vi "PROBE INV SETTING.vi"(8 "INV / NON INV":enum16{"NON INV", "INV"}(ring), 10 "CH":enum16{"CH 1", "CH 2", "CH 3", "CH 4"}(ring), 11 "VISA TSD2014B":refnum<visa-resource-name>="USB0::0x0699::0x0368::C020278::INSTR") -> ()   [LabVIEW 2011]
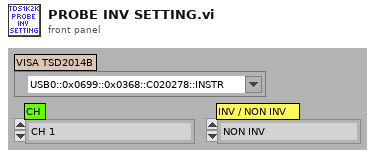
[diagram p1: front panel]
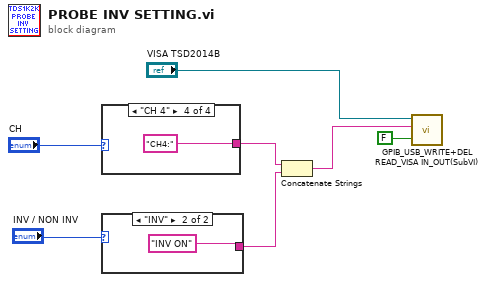
[diagram p0: block diagram]
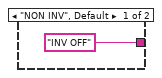
[diagram p2: hidden frame]
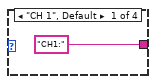
[diagram p3: hidden frame]
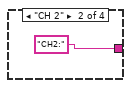
[diagram p4: hidden frame]
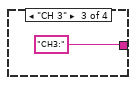
[diagram p5: hidden frame]
diagram:
  n1 = case shown="\"CH 4\"" "CH" {
    tunnel: ["CH1:" "CH2:" "CH3:" "CH4:"] -> w3
    frame "CH 1", Default {
    }
    frame "CH 2" {
    }
    frame "CH 3" {
    }
    frame "CH 4" {
    }
  }
  n2 = case shown="\"INV\"" "INV / NON INV" {
    tunnel: ["INV OFF" "INV ON"] -> w2
    frame "NON INV", Default {
    }
    frame "INV" {
    }
  }
  n3 = Concatenate Strings(w3, w2) -> (w1:string)
  n4 = call "GPIB_USB_WRITE+DEL READ_VISA IN_OUT(SubVI).vi"("VISA resource IN"="VISA TSD2014B", "GPIB/USB WRITE"=w1, 4:FALSE ("READ GPIB")) -> ()  [unwired: 3 in, 3 out]
